vi "Update_Flow_Target.vi"(8 "error in":errorcluster, 10 "Output Flow Rate Target (Automated Test)":dbl=0.76 caption="Output Flow Target (Automated Test)", 11 "Modbus":refnum<queue>) -> (0 "error out":errorcluster)   [LabVIEW 2020]
uses:
  Message Queue/Message Cluster.ctl
  Message Queue/Enqueue Message (Single).vi
  Message Queue/Message Queue.lvlib
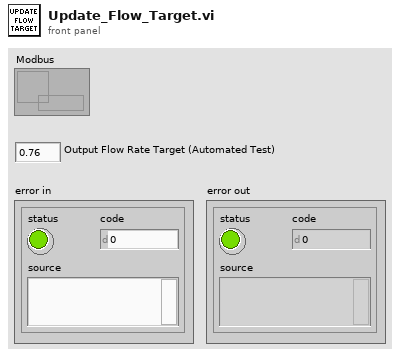
[diagram p1: front panel]
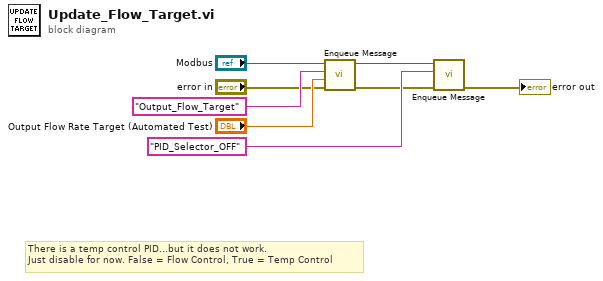
[diagram p0: block diagram]
diagram:
  # "There is a temp control PID...but it does not work.\nJust disable for now. False = Flow Control, True = Temp Control"
  n1 = call-poly "Enqueue Message.vi"("error in (no error)"="error in", "Message Data"="Output Flow Rate Target (Automated Test)", "Message"="Output_Flow_Target", "Message Queue"="Modbus") -> ("error out"=w6:errorcluster, "dup Message Queue"=w7:refnum<queue>)  [unwired: 6 in]
  n2 = call-poly "Enqueue Message.vi"("error in (no error)"=w6, "Message"="PID_Selector_OFF", "Message Queue"=w7) -> ("error out"=→"error out":errorcluster)  [unwired: 7 in, 1 out]
